vi "DAQ_Network-Stream_Reader-Writer.vi"(8 "DAQ ID":i32, 9 "CTR Endpoint":string="CTR001", 10 "DAQ IP Addr":string, 11 "CTR IP Addr":string) -> (0 "//CTR IP Addr:CTR000/DAQ000-Data":string, 1 "//DAQ IP Addr:DAQ000/DAQ000-Data":string, 2 "//CTR IP Addr:CTR000/DAQ000-Control":string, 3 "//DAQ IP Addr:DAQ000/DAQ000-Control":string)   [LabVIEW 2024]
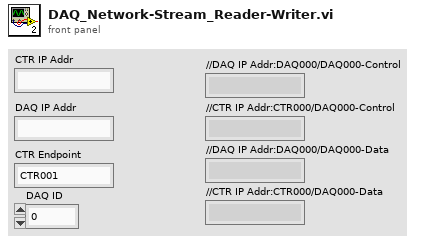
[diagram p1: front panel]
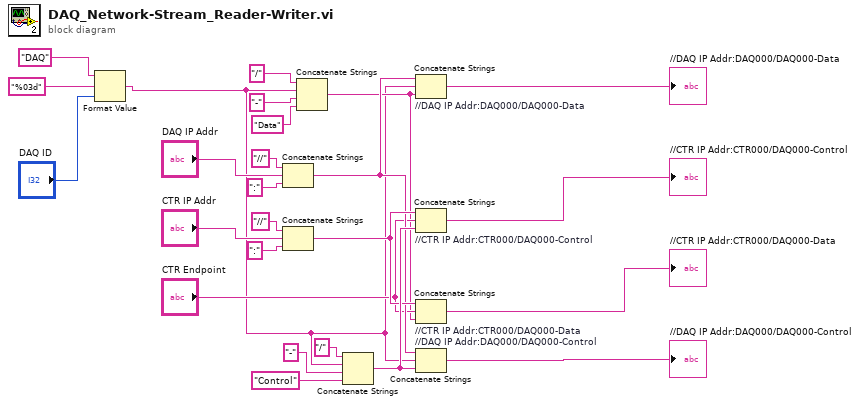
[diagram p0: block diagram]
diagram:
  n1 = Format Value(string ("")="DAQ", format string="%03d", value (0)="DAQ ID") -> (output string=w4:string)
  n2 = Concatenate Strings("//" ("string"), "DAQ IP Addr", ":" ("string")) -> (w9:string)
  n3 = Concatenate Strings("//" ("string"), "CTR IP Addr", ":" ("string")) -> (w10:string)
  n4 = Concatenate Strings("/" ("string"), w4, "-" ("string"), "Data" ("string")) -> (w7:string)
  n5 = Concatenate Strings("/" ("string"), w4, "-" ("string"), "Control" ("string")) -> (w21:string)
  n6 = Concatenate Strings "//DAQ IP Addr:DAQ000/DAQ000-Data"(w9, w4, w7) -> (→"//DAQ IP Addr:DAQ000/DAQ000-Data":string)
  n7 = Concatenate Strings "//CTR IP Addr:CTR000/DAQ000-Control"(w10, "CTR Endpoint", w21) -> (→"//CTR IP Addr:CTR000/DAQ000-Control":string)
  n8 = Concatenate Strings "//CTR IP Addr:CTR000/DAQ000-Data"(w10, "CTR Endpoint", w7) -> (→"//CTR IP Addr:CTR000/DAQ000-Data":string)
  n9 = Concatenate Strings "//DAQ IP Addr:DAQ000/DAQ000-Control"(w9, w4, w21) -> (→"//DAQ IP Addr:DAQ000/DAQ000-Control":string)
